vi "Contador2_DAQ.vi"() -> ()   [LabVIEW 2024]
panel:
  out "Contador":dbl
  in  "stop":bool
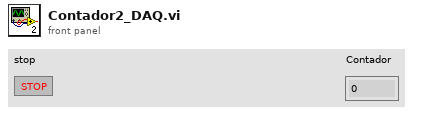
[diagram p1: front panel]
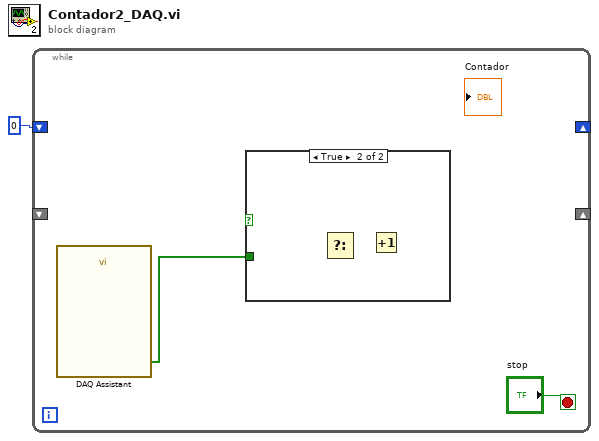
[diagram p0: block diagram]
diagram:
  n1 = while {
    shift-right: _ -> [_]
    shift-left: 0 -> [_]
    shift-right: _ -> [_]
    shift-left: _ -> [_]
    stop <- "stop" stop-if-true
    n2 = call "DAQ Assistant"() -> ("data"=w2:bool[])  [unwired: 17 in, 2 out]
    n3 = case shown="True" {
      selector: _ -> [_ _]
      tunnel: w2 -> [_ _]
      frame False {
      }
      frame True {
        n4 = Select() -> ()  [unwired: 3 in, 1 out]
        n5 = Increment() -> ()  [unwired: 1 in, 1 out]
      }
    }
  }
